vi "Create - Time Stamp is Current Time.vi"() -> ()   [LabVIEW 2013, in "JUnit XML Tests.lvlib" / "Test Suite.lvlib"]
uses:
  Test Suite.lvlib
  JUnit XML/Test Suite/Test Suite.lvclass/Test Suite.ctl
  JUnit XML/Test Suite/Read Timestamp.vi
  <vilib>/addons/_JKI Toolkits/Caraya/classes/Assert/Assert Less Or Equal_Variant.vi
  <vilib>/addons/_JKI Toolkits/Caraya/classes/Assert/Assert Greater Or Equal_Variant.vi
  JUnit XML/Test Suite/Test Suite.lvclass
  <vilib>/addons/_JKI Toolkits/Caraya/classes/Assert/Assert.lvclass
  <vilib>/addons/_JKI Toolkits/Caraya/classes/Test/Test.lvclass
panel:
  out "error out":errorcluster
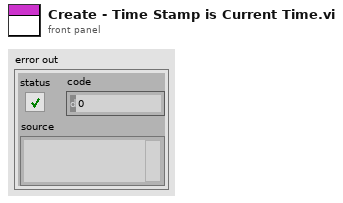
[diagram p1: front panel]
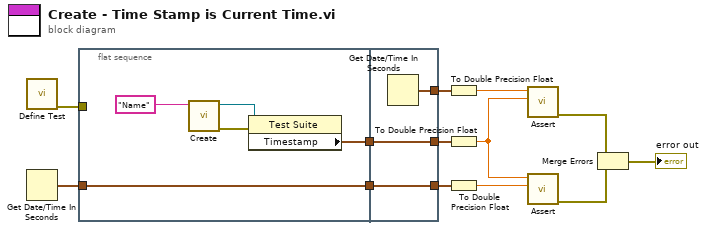
[diagram p0: block diagram]
diagram:
  n1 = call <vilib>:"Define Test.vi"() -> ("error out"=w6:errorcluster)  [unwired: 10 in, 1 out]
  n2 = Get Date/Time In Seconds() -> (seconds since 1Jan1904=w12:timestamp)
  n3 = flat-sequence {
    tunnel: [w16] -> w13
    tunnel: w12 -> [w16]
    tunnel: [w15] -> w11
    tunnel: w6 -> [_]
    tunnel: [w21] -> w5
    tunnel: w13 -> [w21]
    tunnel: [w20] -> w4
    tunnel: w11 -> [w20]
    tunnel: [w19] -> w10
    frame #0 {
      n4 = call "Create.vi"("Name"="Name" ("Package")) -> ("error out"=w18:errorcluster, "Test Suite"=w17:refnum<class "Test Suite.lvclass">)  [unwired: 9 in]
      n5 = property on="Property Node" class="Test Suite"(reference=w17, error in=w18) -> ("Timestamp"=w15:timestamp)  [unwired: 2 out]
    }
    frame #1 {
      n6 = Get Date/Time In Seconds() -> (seconds since 1Jan1904=w19:timestamp)
    }
  }
  n7 = To Double Precision Float(number=w10) -> (double precision float=w3:dbl)
  n8 = To Double Precision Float(number=w4) -> (double precision float=w1:dbl)
  n9 = To Double Precision Float(number=w5) -> (double precision float=w2:dbl)
  n10 = call-poly <vilib>:"Assert.vi"("Actual"=w1, "Expected"=w3) -> ("error out"=w8:errorcluster)  [unwired: 8 in, 1 out]
  n11 = call-poly <vilib>:"Assert.vi"("Actual"=w2, "Expected"=w1) -> ("error out"=w9:errorcluster)  [unwired: 8 in, 1 out]
  n12 = Merge Errors(w8, w9) -> (→"error out":errorcluster)
